vi "net方法-启动模拟器引用.vi"(10 "端口号":u16, 11 "面板VI引用":refnum<vi>) -> (2 "错误输出":errorcluster)   [LabVIEW 2017]
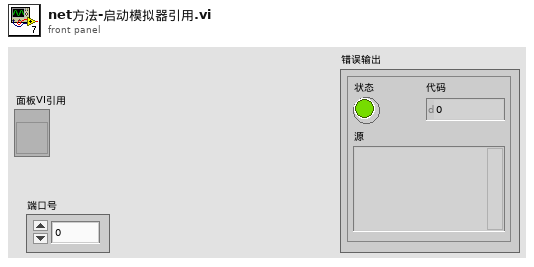
[diagram p1: front panel]
types:
  T1 = enum32{"Invalid", "Standard", "Closed", "Hidden", "Minimized", "Maximized"}
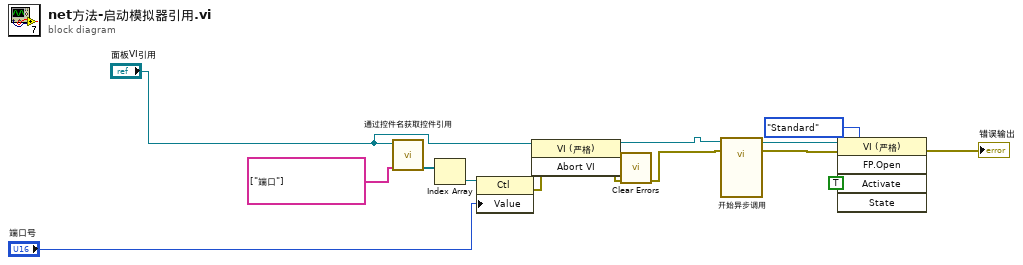
[diagram p0: block diagram]
diagram:
  n1 = call "通过控件名获取控件引用.vi"("控件名数组"=string[] ["端口"], "VI引用"="面板VI引用") -> ("控件引用输出"=w13:refnum<vi>[])  [unwired: 7 in, 2 out]
  n2 = Index Array(array=w13) -> (element=w12:refnum<vi>)  [unwired: 1 in]
  n3 = property class="Ctl"(reference=w12, "Value"="端口号") -> (error out=w10:errorcluster)  [unwired: 1 in, 1 out]
  n4 = invoke class="VI (严格)" method="Abort VI"(reference="面板VI引用", error in=w10) -> (reference out=w5:refnum<vi>, error out=w9:errorcluster)  [unwired: 1 in, 1 out]
  n5 = call <vilib>:"Clear Errors.vi"("error in (no error)"=w9) -> ("error out"=w3:errorcluster)  [unwired: 5 in, 1 out]
  n6 = call-by-ref "开始异步调用"(reference=w5, error in=w3) -> (reference out=w4:refnum<vi>, error out=w2:errorcluster)  [unwired: 12 in]
  n7 = invoke class="VI (严格)" method="FP.Open"(reference=w4, error in=w2, "Activate"=TRUE ("激活？"), "State"=T1."Standard" ("状态")) -> (error out=→"错误输出":errorcluster)  [unwired: 1 in, 4 out]
